vi "stackedSecuence.vi"() -> ()   [LabVIEW 2020]
panel:
  out "Thermometer 4":u8(slide) scale=0.0..100.0
  out "Thermometer 3":u8(slide) scale=0.0..100.0
  out "Thermometer 2":u8(slide) scale=0.0..100.0
  out "Thermometer":u8(slide) scale=0.0..100.0
  # "Stacked Secuence"
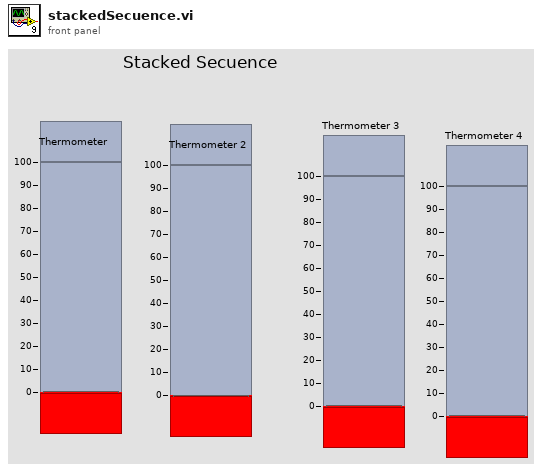
[diagram p1: front panel]
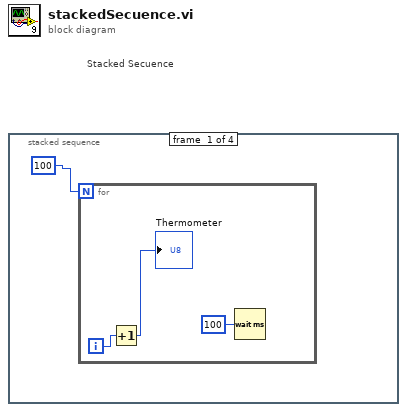
[diagram p0: block diagram]
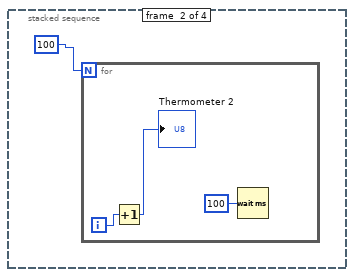
[diagram p2: hidden frame]
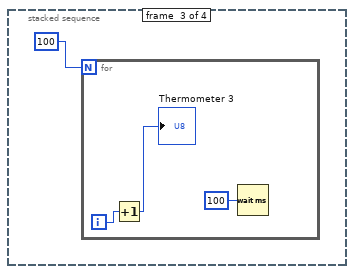
[diagram p3: hidden frame]
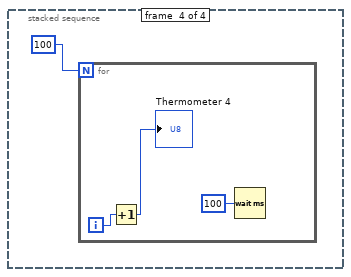
[diagram p4: hidden frame]
diagram:
  # "Stacked Secuence"
  n1 = stacked-sequence {
    frame #0 {
      n2 = for {
        N: 100 -> [_]
        i -> [w4]
        n3 = Increment(x=w4) -> (x+1=→"Thermometer":i32)
        n4 = Wait (ms)(milliseconds to wait=u32 100) -> ()  [unwired: 1 out]
      }
    }
    frame #1 {
      n5 = for {
        N: 100 -> [_]
        i -> [w8]
        n6 = Increment(x=w8) -> (x+1=→"Thermometer 2":i32)
        n7 = Wait (ms)(milliseconds to wait=u32 100) -> ()  [unwired: 1 out]
      }
    }
    frame #2 {
      n8 = for {
        N: 100 -> [_]
        i -> [w12]
        n9 = Increment(x=w12) -> (x+1=→"Thermometer 3":i32)
        n10 = Wait (ms)(milliseconds to wait=u32 100) -> ()  [unwired: 1 out]
      }
    }
    frame #3 {
      n11 = for {
        N: 100 -> [_]
        i -> [w16]
        n12 = Increment(x=w16) -> (x+1=→"Thermometer 4":i32)
        n13 = Wait (ms)(milliseconds to wait=u32 100) -> ()  [unwired: 1 out]
      }
    }
  }
